vi "Desktop Execution - Strip Chart SubVI.vi"(11 "Numeric":i32=2) -> ()   [LabVIEW 2023]
doc: "This subVI generates events for the <B>Desktop Execution Trace Toolkit</B> to capture."
panel:
  out "i":i32
  in  "Boolean":bool=TRUE
  out "Waveform Chart":dbl(graph)
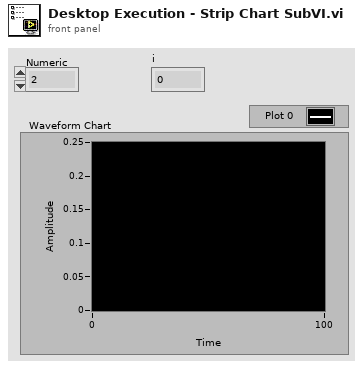
[diagram p1: front panel]
types:
  T1 = enum16{"open", "replace", "create", "open or create", "replace or create", "replace or create with confirmation"}
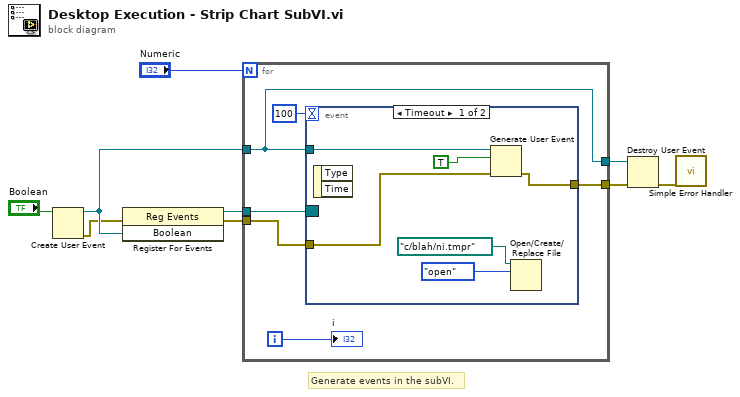
[diagram p0: block diagram]
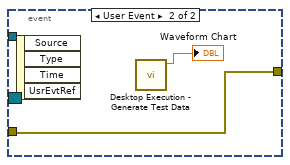
[diagram p2: hidden frame]
diagram:
  # "Generate events in the subVI."
  n1 = Create User Event(user event datatype="Boolean") -> (user event=w7:refnum<user-event>, error out=w2:errorcluster)  [unwired: 1 in]
  n2 = register-events(error in=w2, w7) -> (reference out=w5:refnum<event-registration>, error out=w4:errorcluster)  [unwired: 1 in]
  n3 = for {
    N: "Numeric" -> [_]
    tunnel: w5 -> [w14]
    tunnel: w7 -> [w13]
    tunnel: [w13] -> w6
    tunnel: w4 -> [w12]
    tunnel: [w11] -> w3
    i -> [w10]
    n4 = event shown="[0] Timeout" {
      selector: w14 -> [_ _]
      dyn-events: _ -> [_ _]
      timeout: 100 -> [_ _]
      tunnel: w13 -> [w21 _]
      tunnel: w12 -> [w17 w22]
      tunnel: [w16 w22] -> w11
      event Timeout {
        n5 = event-data() -> ()  [unwired: 3 out]
        n6 = Generate User Event(user event=w21, event data cluster=TRUE ("event data"), error in=w17) -> (error out=w16:errorcluster)  [unwired: 1 in, 1 out]
        n7 = Open/Create/Replace File(file path (use dialog)=path "c:/blah/ni.tmpr", operation (0:open)=T1."open") -> ()  [unwired: 1 in, 6 out]
      }
      event User Event {
        n8 = event-data() -> ()  [unwired: 5 out]
        n9 = call "Desktop Execution - Generate Test Data.vi"() -> ("Random Number"=→"Waveform Chart":dbl)  [unwired: 11 out]
      }
    }
    "i" <- w10
  }
  n10 = Destroy User Event(user event=w6, error in=w3) -> (error out=w1:errorcluster)
  n11 = call <vilib>:"Simple Error Handler.vi"("error in (no error)"=w1) -> ()  [unwired: 4 in, 5 out]
